vi "etlCalibration.vi"(1 "mode":u16(ring) items=["V to dpt", "dpt to V"], 2 "in":dbl) -> (0 "out":dbl)   [LabVIEW 2017]
uses:
  globalDevices.vi
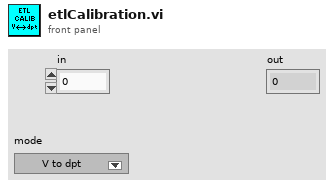
[diagram p1: front panel]
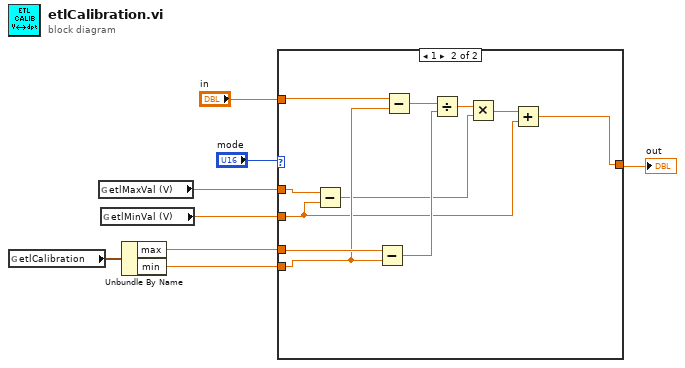
[diagram p0: block diagram]
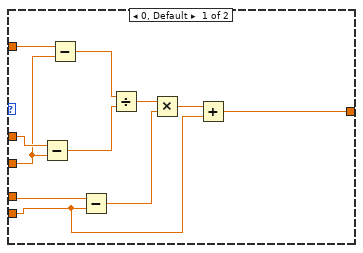
[diagram p2: hidden frame]
diagram:
  n1 = global read "globalDevices.vi" "etlCalibration"() -> (w6:cluster{"min":dbl, "max":dbl})
  n2 = global read "globalDevices.vi" "etlMaxVal (V)"() -> (w5:dbl)
  n3 = global read "globalDevices.vi" "etlMinVal (V)"() -> (w4:dbl)
  n4 = Unbundle By Name(w6) -> ("max"=w3:dbl, "min"=w2:dbl)
  n5 = case shown="1" "mode" {
    tunnel: "in" -> [w17 w28]
    tunnel: w5 -> [w18 w29]
    tunnel: w4 -> [w16 w21]
    tunnel: w3 -> [w19 w30]
    tunnel: w2 -> [w10 w27]
    tunnel: [w9 w20] -> w1
    frame 0, Default {
      n6 = Subtract(x=w18, y=w16) -> (x-y=w14:dbl)
      n7 = Subtract(x=w17, y=w16) -> (x-y=w15:dbl)
      n8 = Subtract(x=w19, y=w10) -> (x-y=w12:dbl)
      n9 = Divide(x=w15, y=w14) -> (x/y=w13:dbl)
      n10 = Multiply(x=w13, y=w12) -> (x*y=w11:dbl)
      n11 = Add(x=w11, y=w10) -> (x+y=w9:dbl)
    }
    frame 1 {
      n12 = Subtract(x=w29, y=w21) -> (x-y=w23:dbl)
      n13 = Subtract(x=w30, y=w27) -> (x-y=w25:dbl)
      n14 = Subtract(x=w28, y=w27) -> (x-y=w26:dbl)
      n15 = Divide(x=w26, y=w25) -> (x/y=w24:dbl)
      n16 = Multiply(x=w24, y=w23) -> (x*y=w22:dbl)
      n17 = Add(x=w22, y=w21) -> (x+y=w20:dbl)
    }
  }
  "out" <- w1
